vi "On Navigation Starting.vi"(8 "error in (no error)":errorcluster, 10 "Nav Started Event":T1, 11 "WebView2 Event Filter Interface in":refnum<class "WebView2 Event Filter Interface.lvclass">) -> (0 "error out":errorcluster, 2 "Cancel":bool)   [LabVIEW 2025, in "WebView2.lvlib" / "WebView2 Event Filter Interface.lvclass"]
uses:
  WebView2 Event Filter Interface.lvclass
  WebView2 Control Object/Navigation Start Event Data.ctl
  WebView2 Control Object/WebView2 Control.lvclass
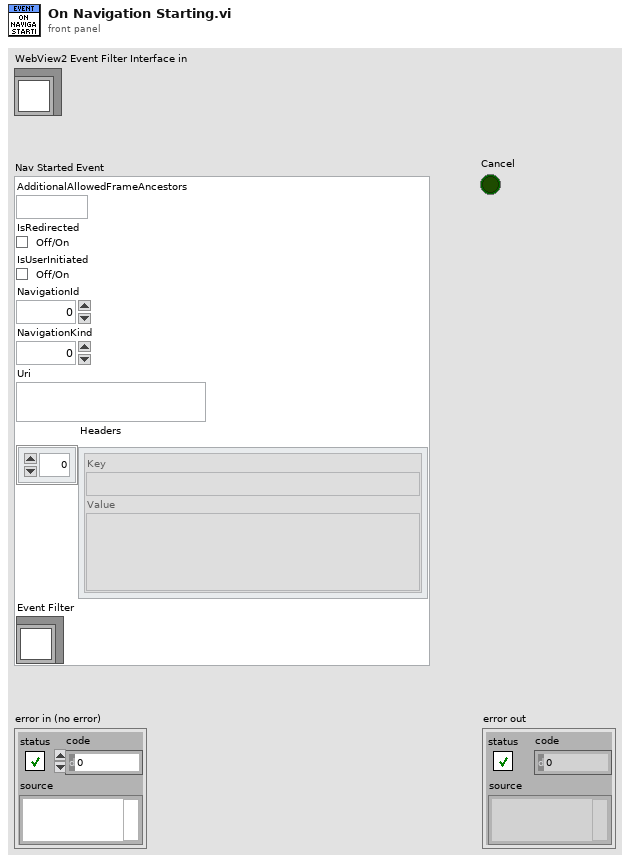
[diagram p1: front panel]
types:
  T1 = typedef "WebView2.lvlib/WebView2 Control.lvclass/Navigation Start Event Data.ctl" = cluster{"AdditionalAllowedFrameAncestors":string, "IsRedirected":bool, "IsUserInitiated":bool, "NavigationId":u64, "NavigationKind":i32, "Uri":string, "Headers":cluster{"Key":string, "Value":string}[], "Event Filter":refnum<class "WebView2 Event Filter Interface.lvclass">}
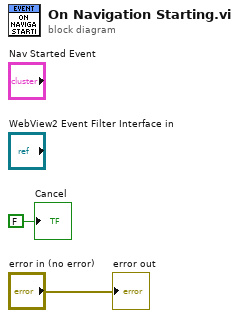
[diagram p0: block diagram]
diagram:
  "error out" <- "error in (no error)"
  "Cancel" <- FALSE ("Cancel")
